vi "YJoystick.vi"(11 "Left Y-Axis":dbl) -> (2 "Left Motor":dbl, 3 "Right Motor":dbl)   [LabVIEW 2013]
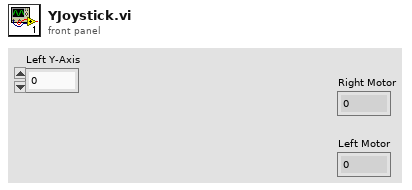
[diagram p1: front panel]
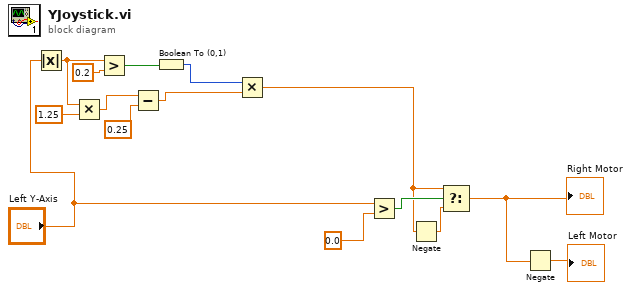
[diagram p0: block diagram]
diagram:
  n1 = Absolute Value(x="Left Y-Axis") -> (abs(x)=w14:dbl)
  n2 = Multiply(x=w14, y=1.25) -> (x*y=w12:dbl)
  n3 = Greater?(x=w14, y=0.2) -> (0:w10:bool)
  n4 = Subtract(x=w12, y=0.25) -> (x-y=w8:dbl)
  n5 = Boolean To (0,1)(Boolean=w10) -> (0, 1=w9:i16)
  n6 = Multiply(x=w9, y=w8) -> (x*y=w4:dbl)
  n7 = Greater?(x="Left Y-Axis", y=0.0) -> (0:w6:bool)
  n8 = Negate(x=w4) -> (-x=w3:dbl)
  n9 = Select(t=w4, s=w6, f=w3) -> (s? t:f=w2:dbl)
  "Right Motor" <- w2
  n10 = Negate(x=w2) -> (-x=→"Left Motor":dbl)
